vi "SwerveModuleOdometry2.vi"(4 "Robot Heading(deg)":dbl, 5 "Module Fault":bool, 6 "Wheel Distance (in)":dbl, 7 "Wheel Azimuth (deg)":dbl, 8 "Actual Shifter State":T1(ring), 9 "Velocity (ft/s)":dbl) -> (0 "Delta Y (in)":dbl, 1 "Delta X (in)":dbl, 2 "Velocity Y (ft/s)":dbl, 3 "Velocity X (ft/s)":dbl)   [LabVIEW 2019]
doc: "This VI calculates the field-centric delta odometry and velocity vectors for a single swerve module."
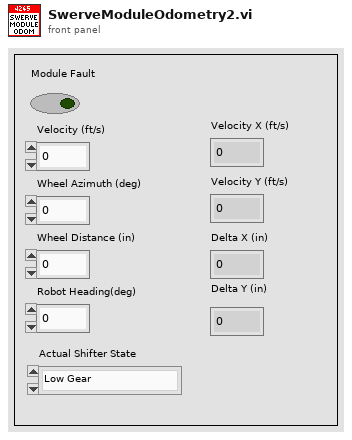
[diagram p1: front panel]
types:
  T1 = enum16{"Low Gear", "High Gear", "Transiting", "Unknown", "Force Low Gear"}
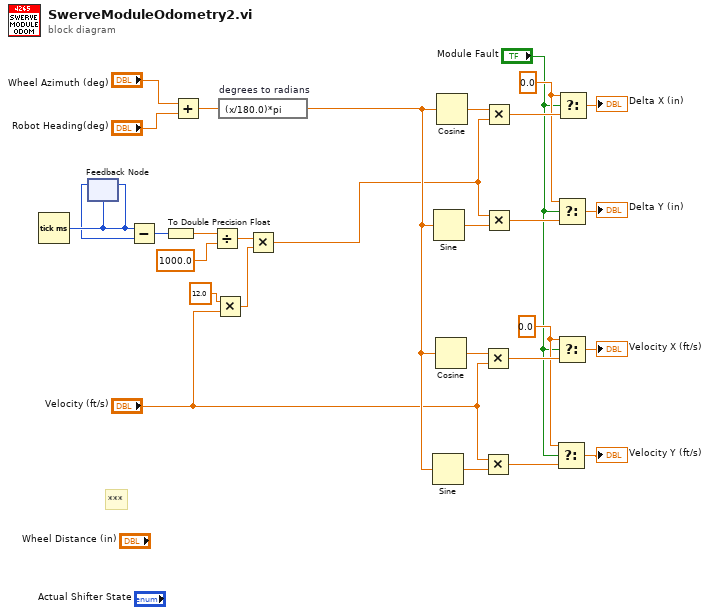
[diagram p0: block diagram]
diagram:
  w15 = 0.0 ("t")
  w20 = 0.0 ("t")
  # "***"
  n1 = Tick Count (ms)() -> (millisecond timer value=w10:u32)
  n2 = feedback-in #1(w10) -> ()
  n3 = feedback #1(w10) -> (w9:u32)
  n4 = Subtract(x=w10, y=w9) -> (x-y=w8:u32)
  n5 = To Double Precision Float(number=w8) -> (double precision float=w7:dbl)
  n6 = Add(x="Wheel Azimuth (deg)", y="Robot Heading(deg)") -> (x+y=w25:dbl)
  n7 = Divide(x=w7, y=1000.0) -> (x/y=w3:dbl)
  n8 = Multiply(x=12.0 ("y"), y="Velocity (ft/s)") -> (x*y=w2:dbl)
  n9 = expression code="(x/180.0)*pi" "degrees to radians"(w25) -> (w11:dbl)
  n10 = Multiply(x=w3, y=w2) -> (x*y=w1:dbl)
  n11 = Sine(x=w11) -> (sin(x)=w19:dbl)
  n12 = Sine(x=w11) -> (sin(x)=w27:dbl)
  n13 = Cosine(x=w11) -> (cos(x)=w18:dbl)
  n14 = Cosine(x=w11) -> (cos(x)=w26:dbl)
  n15 = Multiply(x=w18, y="Velocity (ft/s)") -> (x*y=w17:dbl)
  n16 = Multiply(x="Velocity (ft/s)", y=w19) -> (x*y=w16:dbl)
  n17 = Multiply(x=w26, y=w1) -> (x*y=w22:dbl)
  n18 = Multiply(x=w1, y=w27) -> (x*y=w21:dbl)
  n19 = Select(t=w15, s="Module Fault", f=w16) -> (s? t:f=→"Velocity Y (ft/s)":dbl)
  n20 = Select(t=w20, s="Module Fault", f=w21) -> (s? t:f=→"Delta Y (in)":dbl)
  n21 = Select(t=w15, s="Module Fault", f=w17) -> (s? t:f=→"Velocity X (ft/s)":dbl)
  n22 = Select(t=w20, s="Module Fault", f=w22) -> (s? t:f=→"Delta X (in)":dbl)
